vi "Teleop - Multi Sample Average (SubVI).vi"(10 "Input":dbl, 11 "Samples to average":i32) -> (3 "Output":dbl)   [LabVIEW 2019]
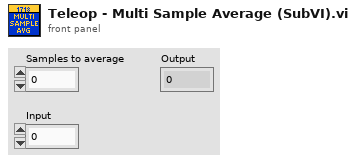
[diagram p1: front panel]
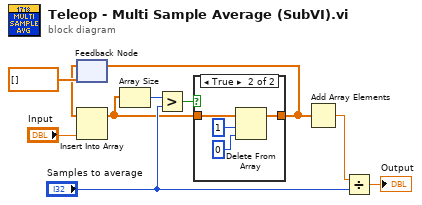
[diagram p0: block diagram]
diagram:
  n1 = feedback #1(dbl[] []) -> (w1:dbl[])
  n2 = Insert Into Array(array=w1, new element="Input") -> (w5:dbl[])  [unwired: 1 in]
  n3 = Array Size(array=w5) -> (size(s)=w3:i32)
  n4 = Greater?(x=w3, y="Samples to average") -> (0:w4:bool)
  n5 = case shown="True" w4 {
    tunnel: w5 -> [w11 w15]
    tunnel: [w11 w14] -> w6
    frame False {
    }
    frame True {
      n6 = Delete From Array(array=w15, length=1, index=0) -> (array with subset deleted=w14:dbl[])  [unwired: 1 out]
    }
  }
  n7 = feedback-in #1(w6) -> ()
  n8 = Add Array Elements(numeric array=w6) -> (sum=w7:dbl)
  n9 = Divide(x=w7, y="Samples to average") -> (x/y=→"Output":dbl)
